vi "Create.vi"(8 "error in (no error)":errorcluster, 11 "Document in":refnum<class "Document.lvclass">) -> (0 "error out":errorcluster, 3 "Document out":refnum<class "Document.lvclass">)   [LabVIEW 2016, in "Document.lvclass"]
uses:
  Document.lvclass
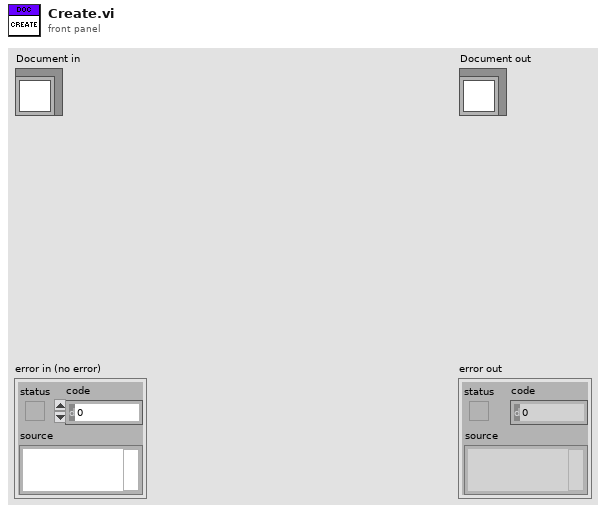
[diagram p1: front panel]
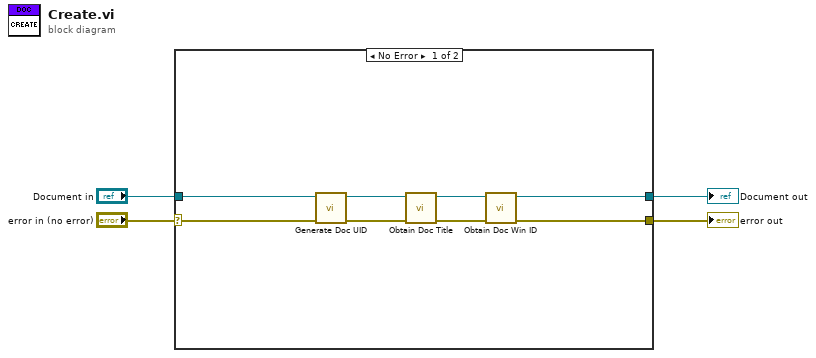
[diagram p0: block diagram]
diagram:
  n1 = case shown="No Error" "error in (no error)" {
    selector: "error in (no error)" -> [w6 w14]
    tunnel: [w5 w14] -> w3
    tunnel: [w9 w13] -> w1
    tunnel: "Document in" -> [w10 w13]
    frame No Error {
      n2 = call-dynamic "Generate Doc UID.vi"("error in (no error)"=w6, "Document in"=w10) -> ("error out"=w8:errorcluster, "Document out"=w12:refnum<class "Document.lvclass">)  [unwired: 8 in]
      n3 = call-dynamic "Obtain Doc Title.vi"("error in (no error)"=w8, "Document in"=w12) -> ("error out"=w7:errorcluster, "Document out"=w11:refnum<class "Document.lvclass">)  [unwired: 8 in]
      n4 = call-dynamic "Obtain Doc Win ID.vi"("error in (no error)"=w7, "Document in"=w11) -> ("error out"=w5:errorcluster, "Document out"=w9:refnum<class "Document.lvclass">)  [unwired: 8 in]
    }
    frame Error {
    }
  }
  "error out" <- w3
  "Document out" <- w1
